vi "TimingInfo.vi"(1 "Get/Set":bool, 2 "Timing Info (input)":T1={"Fs"=1.0, "#s"=10.0} {"#s" format="%.2f"; "Fs" format="%.2f"}) -> (0 "Timing Info (output)":T1={"Fs"=1.0, "#s"=10.0} {"#s" format="%.2f"; "Fs" format="%.2f"})   [LabVIEW 2009]
uses:
  TimingInfo.ctt
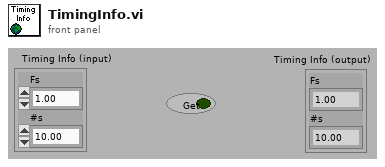
[diagram p1: front panel]
types:
  T1 = typedef "TimingInfo.ctt" = cluster{"Fs":dbl, "#s":dbl}
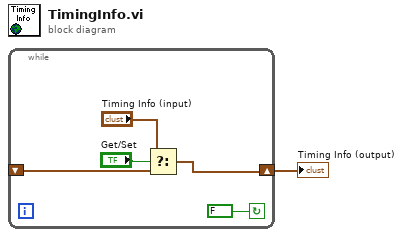
[diagram p0: block diagram]
diagram:
  n1 = while {
    shift-right: [w4] -> w1
    shift-left: _ -> [w5]
    stop <- FALSE continue-if-true
    n2 = Select(t="Timing Info (input)", s="Get/Set", f=w5) -> (s? t:f=w4:T1)
  }
  "Timing Info (output)" <- w1
